vi "todelete.vi"() -> ()   [LabVIEW 2016]
uses:
  <vilib>/Analysis/coordinate.llb/Euler Rotation Order.ctl
  Vision Server/typedef/Target Vector.ctl
  <vilib>/Analysis/coordinate.llb/3D Cartesian Coordinate Rotation (Euler) (Scalar).vi
  <vilib>/Analysis/NI_AALPro.lvlib
  Vision Server/Vision Server.lvclass
panel:
  out "zr":dbl
  out "yr":dbl
  out "xr":dbl
  out "x out":dbl
  out "y out":dbl
  out "z out":dbl
  out "error":i32
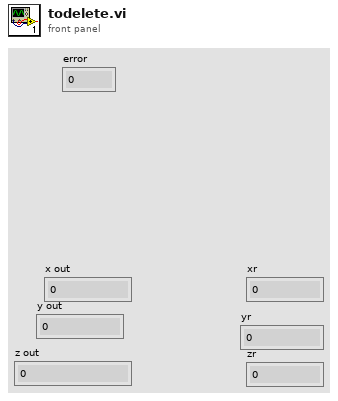
[diagram p1: front panel]
types:
  T1 = typedef "Vision Server.lvclass/Target Vector.ctl" = cluster{"y":dbl, "z":dbl}
  T2 = typedef "NI_AALPro.lvlib/Euler Rotation Order.ctl" = u16
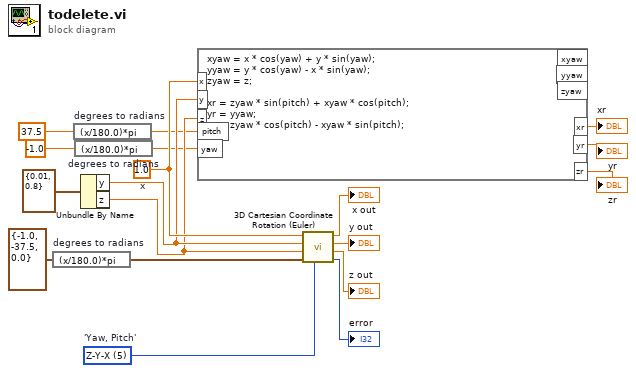
[diagram p0: block diagram]
diagram:
  w18 = T2 5 items=["X-Y-Z", "X-Z-Y", "Y-X-Z", "Y-Z-X", "Z-X-Y", "Z-Y-X", "X-Y-X", "X-Z-X", "Y-X-Y", "Y-Z-Y", "Z-X-Z", "Z-Y-Z"]  # 'Yaw, Pitch'
  w11 = 1.0  # x
  n1 = expression code="(x/180.0)*pi" "degrees to radians"(cluster{"phi":dbl, "theta":dbl, "psi":dbl} {"phi"=-1.0, "theta"=-37.5, "psi"=0.0} ("Euler Angles")) -> (w8:cluster{"phi":dbl, "theta":dbl, "psi":dbl})
  n2 = expression code="(x/180.0)*pi" "degrees to radians"(37.5 ("input variable")) -> (w2:dbl)
  n3 = expression code="(x/180.0)*pi" "degrees to radians"(-1.0 ("input variable")) -> (w1:dbl)
  n4 = Unbundle By Name(T1 {"y"=0.01, "z"=0.8} ("input cluster")) -> ("y"=w10:dbl, "z"=w9:dbl)
  n5 = formula code="xyaw = x * cos(yaw) + y * sin(yaw);\nyyaw = y * cos(yaw) - x * sin(yaw);\nzyaw = z;\n\nxr = zyaw * sin(pitch) + xyaw * cos(pitch);\nyr = yyaw;\nzr = zyaw * cos(pitch) - xyaw * sin(pitch);"("x"=w11, "y"=w10, "z"=w9, "pitch"=w2, "yaw"=w1) -> ("xr"=→"xr":dbl, "yr"=→"yr":dbl, "zr"=→"zr":dbl)  [unwired: 3 out]
  n6 = call-poly <vilib>:"3D Cartesian Coordinate Rotation (Euler).vi"("rotation order"=w18, "Euler Angles"=w8, "z"=w9, "y"=w10, "x"=w11) -> ("error"=→"error":i32, "z out"=→"z out":dbl, "y out"=→"y out":dbl, "x out"=→"x out":dbl)  [unwired: 3 in]
